vi "getLutApplied.vi"(8 "error":errorcluster, 10 "axis":i32, 11 "connection ID":refnum<k5>) -> (0 "error out":errorcluster, 1 "apply":bool, 2 "axis_out":i32, 3 "connection ID out":refnum<k5>)   [LabVIEW 2016, in "sen_api.lvlib"]
doc: "Returns whether a LUT is applied or not for a specific measurement axis."
uses:
  sen_api.lvlib
panel:
  out "jsonRespIn":string
  out "JSON-response":string="{\"jsonrpc\":\"2.0\",\"method\":\"\",\"params\":[5,1.245,true,\"name\"],\"id\":\"1\"}"
  out "JSON request":string
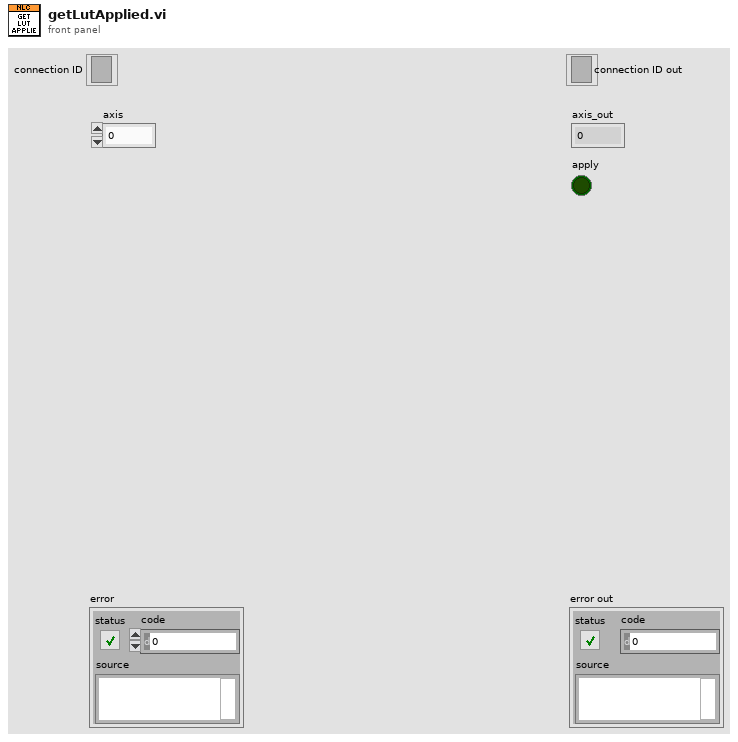
[diagram p1: front panel]
types:
  T1 = cluster{"jsonrpc":string, "method":string, "params":string[], "id":string, "api":i32, "pid":string}
  T2 = enum16{"Standard", "Buffered", "CRLF", "Immediate"}
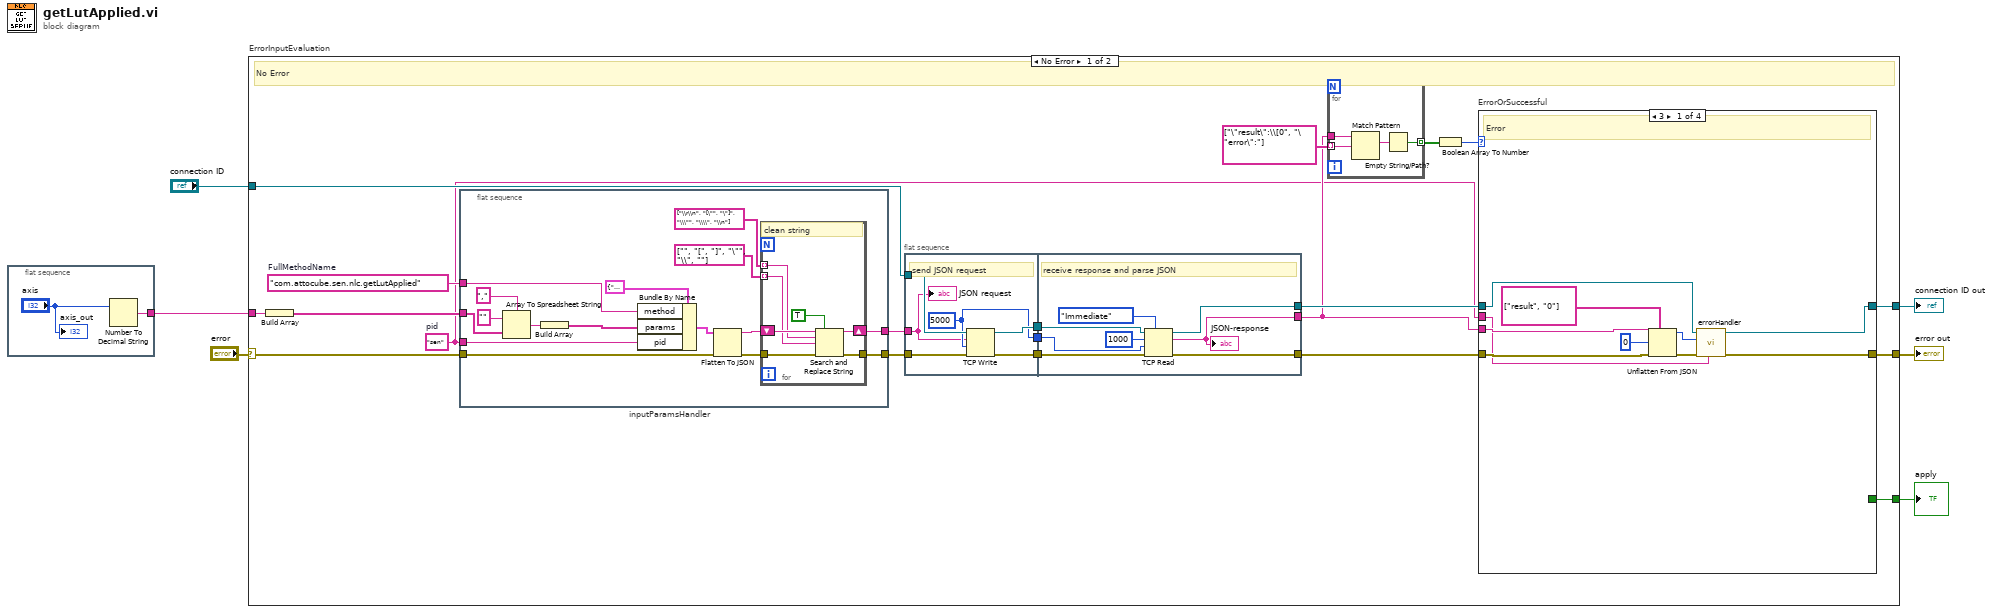
[diagram p0: block diagram]
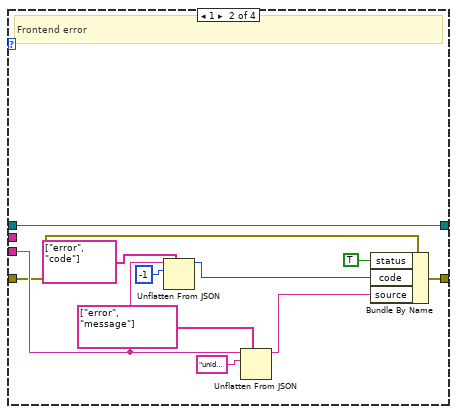
[diagram p2: hidden frame]
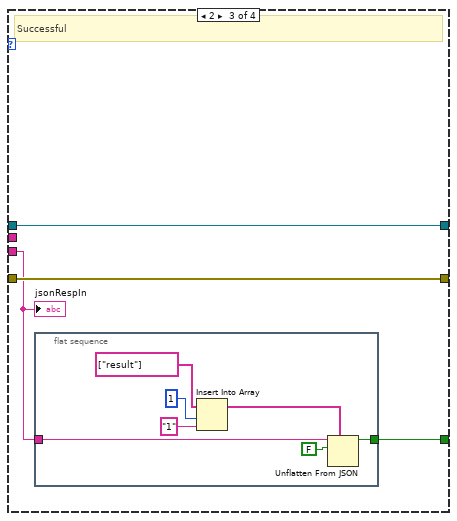
[diagram p3: hidden frame]
diagram:
  n1 = flat-sequence "in_axis" {
    tunnel: [w8] -> w2
    frame #0 {
      n2 = Number To Decimal String(number="axis") -> (decimal integer string=w8:string)  [unwired: 1 in]
      "axis_out" <- "axis"
    }
  }
  n3 = case "ErrorInputEvaluation" shown="No Error" "error" {
    selector: "error" -> [w15 w104]
    tunnel: "connection ID" -> [w25 w105]
    tunnel: [w17 w104] -> w5
    tunnel: [w18 w105] -> w4
    tunnel: w2 -> [w10 _]
    tunnel: [w9 _] -> w1
    frame No Error {
      w11 = "sen"  # pid
      w16 = "com.attocube.sen.nlc.getLutApplied"  # FullMethodName
      # "No Error"
      n4 = Build Array ("ParametersArrayString")(w10) -> (w14:string[])
      n5 = flat-sequence "inputParamsHandler" {
        tunnel: [w32] -> w13
        tunnel: w14 -> [w39]
        tunnel: w15 -> [w37]
        tunnel: [w34] -> w12
        tunnel: w16 -> [w40]
        tunnel: w11 -> [w29]
        frame #0 {
          n6 = Array To Spreadsheet String(delimiter (Tab)=",", array=w39, 3:"" ("format string")) -> (spreadsheet string=w42:string)
          n7 = Build Array "Build Array"(w42) -> (w38:string[])
          n8 = Bundle By Name(cluster=T1 {"jsonrpc"="2.0", "method"="com.attocube.amc.res.setRESReadOutFreq", "params"=[], "id"="1", "api"=2, "pid"=""}, "method"=w40, "params"=w38, "pid"=w29) -> (w41:T1)
          n9 = Flatten To JSON(anything=w41, error in (no error)=w37) -> (JSON string=w33:string, 11:w35:errorcluster)  [unwired: 1 in]
          n10 = for {
            tunnel: string[] ["\\r\\n", "[\"", "\"]", "\\\"", "\\\\", "\\n"] ("search string") -> [w48] mode=indexing
            tunnel: string[] ["", "[", "]", "\"", "\\", ""] ("replace string (\"\")") -> [w47] mode=indexing
            shift-right: [w50] -> w32
            shift-left: w33 -> [w49]
            tunnel: w35 -> [w46]
            tunnel: [w45] -> w34
            # "clean string"
            n11 = Search and Replace String(replace all?=TRUE ("replace all? (F)"), input string=w49, search string=w48, replace string=w47, error in=w46) -> (result string=w50:string, error out=w45:errorcluster)  [unwired: 3 in, 2 out]
          }
        }
      }
      n12 = flat-sequence {
        tunnel: w25 -> [w95]
        tunnel: [w93] -> w28
        tunnel: [w94] -> w27
        tunnel: w12 -> [w90]
        tunnel: [w92] -> w26
        tunnel: w13 -> [w91]
        tunnel: [w99] -> w21
        tunnel: w28 -> [w101]
        tunnel: w27 -> [w100]
        tunnel: [w97] -> w20
        tunnel: w26 -> [w98]
        tunnel: [w96] -> w19
        frame #0 {
          w92 = 5000 ("timeout ms (25000)")
          # "send JSON request"
          n13 = TCP Write(connection ID=w95, data in=w91, error in (no error)=w90, 9:w92) -> (connection ID out=w93:refnum<k5>, error out=w94:errorcluster)  [unwired: 1 out]
          "JSON request" <- w91
        }
        frame #1 {
          # "receive response and parse JSON"
          n14 = TCP Read(connection ID=w101, bytes to read=1000, error in (no error)=w100, 7:T2."Immediate" ("mode (standard)"), 9:w98) -> (connection ID out=w99:refnum<k5>, data out=w96:string, error out=w97:errorcluster)
          "JSON-response" <- w96
        }
      }
      n15 = for {
        tunnel: string[] ["\"result\":\\[0", "\"error\":"] ("path") -> [w54] mode=indexing
        tunnel: [w52] -> w23 mode=indexing
        tunnel: w19 -> [w55]
        n16 = Match Pattern(string=w55, regular expression=w54) -> (match substring=w53:string)  [unwired: 1 in, 3 out]
        n17 = Empty String/Path?(string/path=w53) -> (empty?=w52:bool)
      }
      n18 = Boolean Array To Number(Boolean array=w23) -> (number=w22:u32)
      n19 = case "ErrorOrSuccessful" shown="3" w22 {
        tunnel: w19 -> [w59 w68 w78 _]
        tunnel: w21 -> [w63 w66 w80 w89]
        tunnel: [w61 w66 w80 w89] -> w18
        tunnel: [w62 w69 w79 w88] -> w17
        tunnel: w20 -> [w65 w67 w79 w88]
        tunnel: w11 -> [w56 _ _ _]
        tunnel: [_ _ w77 _] -> w9
        frame 3 {
          # "Error"
          n20 = Unflatten From JSON(path=string[] ["result", "0"], JSON string=w59, type and defaults=0, error in (no error)=w65) -> (value=w57:i32, error out=w64:errorcluster)  [unwired: 3 in]
          n21 = call "errorHandler.vi"("pid"=w56, "error in"=w64, "errNbr"=w57, "connection ID"=w63) -> ("error out 2"=w62:errorcluster, "connection ID out"=w61:refnum<k5>)  [unwired: 6 in]
        }
        frame 1 {
          # "Frontend error"
          n22 = Unflatten From JSON(path=string[] ["error", "code"], JSON string=w68, type and defaults=-1) -> (value=w75:i32)  [unwired: 4 in, 1 out]
          n23 = Unflatten From JSON(path=string[] ["error", "message"], JSON string=w68, type and defaults="unidentified error") -> (value=w76:string)  [unwired: 4 in, 1 out]
          n24 = Bundle By Name(cluster=w67, "status"=TRUE, "code"=w75, "source"=w76) -> (w69:errorcluster)
        }
        frame 2 {
          # "Successful"
          n25 = flat-sequence "out_bool" {
            tunnel: w78 -> [w86]
            tunnel: [w81] -> w77
            frame #0 {
              n26 = Insert Into Array "Insert Into Array"(array=string[] ["result"] ("path"), index=1, new element="1" ("idx")) -> (w83:string[])
              n27 = Unflatten From JSON(path=w83, JSON string=w86, type and defaults=FALSE) -> (value=w81:bool)  [unwired: 4 in, 1 out]
            }
          }
          "jsonRespIn" <- w78
        }
        frame Default {
          # "NoResponse"
        }
      }
    }
    frame Error {
      # "Error"
    }
  }
  "error out" <- w5
  "connection ID out" <- w4
  "apply" <- w1
